vi "Set Parameter.vi"(4 "RingText.Text":string, 6 "txtpower":dbl, 7 "txtstepwave":dbl, 8 "error in":errorcluster, 9 "txtstopwave":dbl, 10 "txtstartwave":dbl, 11 "Address Cluster":T1 {"PCU_communcation_method" items=["GPIB", "C232C", "TCPIP", "USB"]; "tsl_communcation_method" items=["GPIB", "C232C", "TCPIP", "USB"]; "MPM_communcation_method" items=["GPIB", "C232C", "TCPIP", "USB"]}) -> (0 "error out":errorcluster, 3 "PDLSTS":refnum<k24>)   [LabVIEW 2017]
uses:
  CTL/Address Cluster.ctl
  D:/test/PDLSTS/LV_PDL_Sample/DLL/InstrumentDLL.dll
  DLL/InstrumentDLL.dll
  D:/test/PDLSTS/LV_PDL_Sample/DLL/STSProcess.dll
  DLL/STSProcess.dll
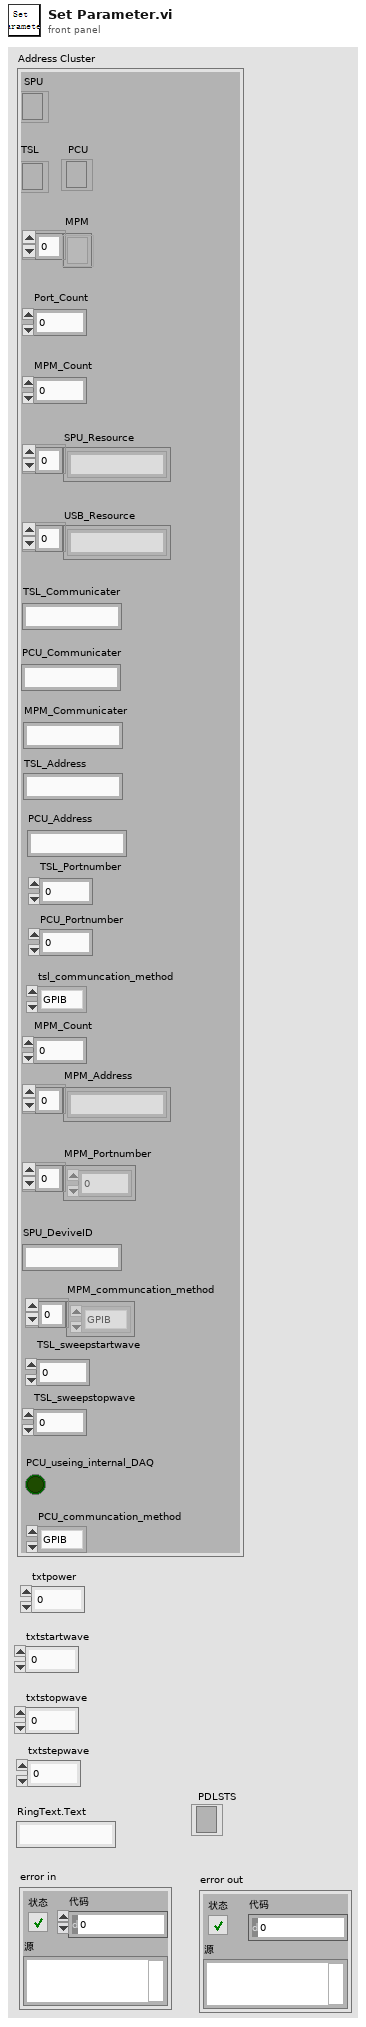
[diagram p1: front panel]
types:
  T1 = typedef "Address Cluster.ctl" = cluster{"SPU":refnum<k24>, "MPM":refnum<k24>[], "Port_Count":dbl, "MPM_Count":dbl, "SPU_Resource":string[], "USB_Resource":string[], "MPM_Communicater":string, "MPM_Count":dbl, "MPM_Address":string[], "MPM_Portnumber":dbl[], "SPU_DeviveID":string, "MPM_communcation_method":i32[], "TSL_sweepstartwave":dbl, "TSL_sweepstopwave":dbl, "TSL_Address":string, "TSL_Communicater":string, "TSL":refnum<k24>, "tsl_communcation_method":i32, "TSL_Portnumber":dbl, "PCU":refnum<k24>, "PCU_Communicater":string, "PCU_Address":string, "PCU_Portnumber":dbl, "PCU_useing_internal_DAQ":bool, "PCU_communcation_method":i32}
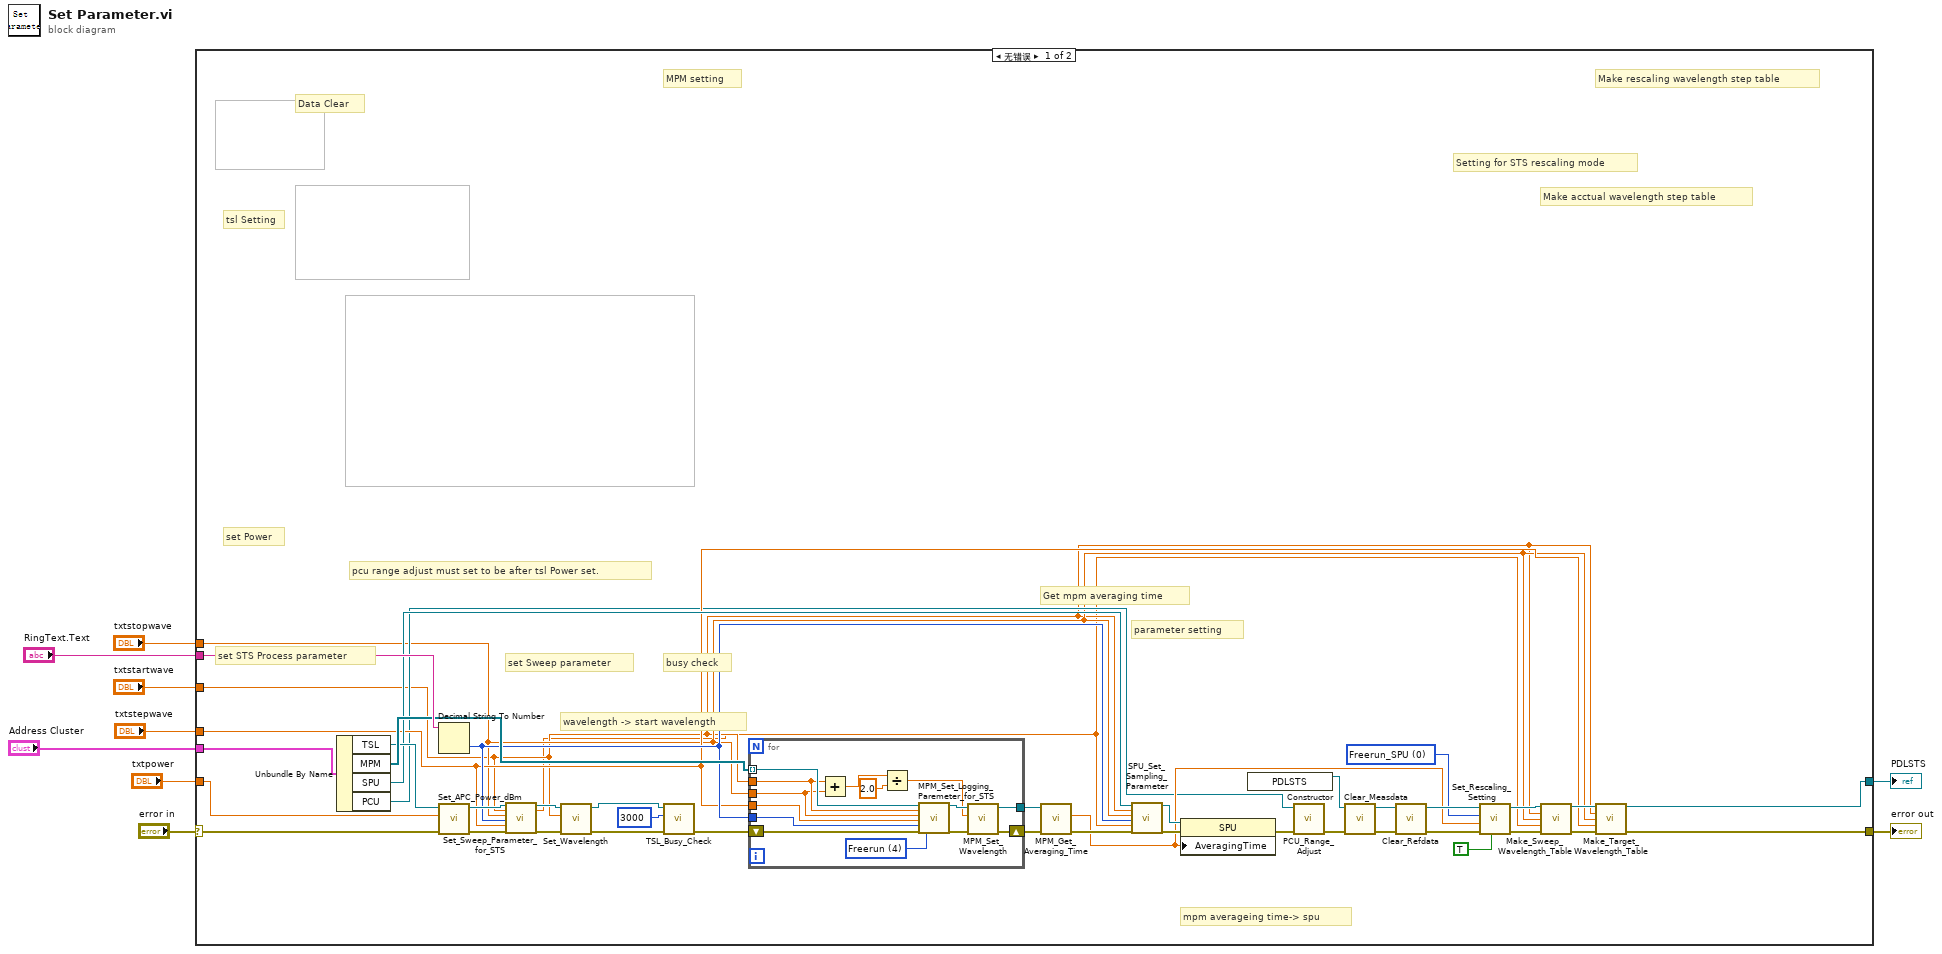
[diagram p0: block diagram]
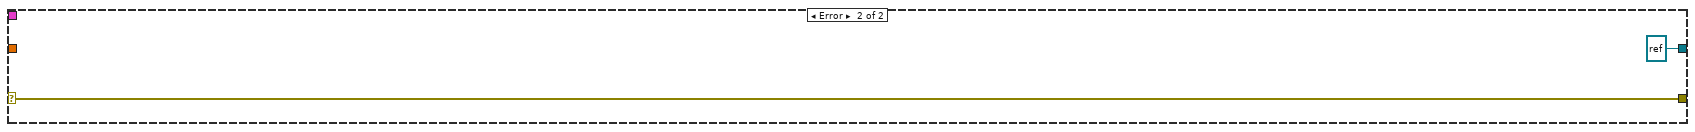
[diagram p2: hidden frame]
diagram:
  n1 = case shown="无错误" "error in" {
    selector: "error in" -> [w47 w67]
    tunnel: "txtstepwave" -> [w22 _]
    tunnel: "RingText.Text" -> [w51 _]
    tunnel: "txtpower" -> [w50 _]
    tunnel: [w13 refnum<k24> refnum ("Reference out")] -> w1
    tunnel: "Address Cluster" -> [w48 _]
    tunnel: [w46 w67] -> w4
    tunnel: "txtstopwave" -> [w12 _]
    tunnel: "txtstartwave" -> [w11 _]
    frame No Error {
      w36 = 0 items=["Freerun_SPU", "Freerun_Referencemodule"] ("mode")
      # "Make rescaling wavelength step table"
      # "Make acctual wavelength step table"
      # "Setting for STS rescaling mode"
      # "Data Clear"
      # "pcu range adjust must set to be after tsl Power set."
      # "mpm averageing time-> spu"
      # "parameter setting"
      # "Get mpm averaging time"
      # "MPM setting"
      # "busy check"
      # "set Sweep parameter"
      # "tsl Setting"
      # "set Power"
      # "set STS Process parameter"
      # "wavelength -> start wavelength"
      n2 = Unbundle By Name(w48) -> ("TSL"=w29:refnum<k24>, "MPM"=w49:refnum<k24>[], "SPU"=w25:refnum<k24>, "PCU"=w17:refnum<k24>)
      n3 = Decimal String To Number(string=w51) -> (number=w23:i32)  [unwired: 2 in, 1 out]
      n4 = call "Set_APC_Power_dBm.vi"(".NET Reference in"=w29, "Setting Power"=w50, "error in (no error)"=w47) -> ("Reference out"=w44:refnum<k24>, "error out"=w45:errorcluster)  [unwired: 6 in]
      n5 = call "Set_Sweep_Parameter_for_STS.vi"(".NET Reference in"=w44, "startwave"=w11, "stopwave"=w12, "speed"=w23, "rescalingstep"=w22, "error in (no error)"=w45) -> ("Reference out"=w43:refnum<k24>, "acctualstep"=w10:dbl, "error out"=w42:errorcluster)  [unwired: 11 in]
      n6 = call "Set_Wavelength.vi"("error in (no error)"=w42, "txtsetwave"=w11, ".NET Reference in"=w43) -> ("error out"=w28:errorcluster, "Reference out"=w21:refnum<k24>)  [unwired: 3 in]
      n7 = call "TSL_Busy_Check.vi"("error in (no error)"=w28, "Wait time(msec)"=3000, ".NET Reference in"=w21) -> ("error out"=w27:errorcluster)  [unwired: 7 in, 1 out]
      n8 = for {
        tunnel: w49 -> [w65] mode=indexing
        tunnel: w11 -> [w56]
        tunnel: w12 -> [w55]
        tunnel: w23 -> [w63]
        tunnel: w22 -> [w61]
        shift-right: [w59] -> w30
        shift-left: w27 -> [w64]
        tunnel: [w58] -> w31
        w62 = 4 items=["ManualRangeConstant", "ManualRangeSweep", "AutoRangeConstant", "AutoRangeSweep", "Freerun"] ("mode")
        n9 = Add(x=w56, y=w55) -> (x+y=w54:dbl)
        n10 = Divide(x=w54, y=2.0) -> (x/y=w52:dbl)
        n11 = call "MPM_Set_Logging_Paremeter_for_STS.vi"(".NET Reference in"=w65, "startwave"=w56, "stopwave"=w55, "wavestep"=w61, "speed"=w63, "error in (no error)"=w64, "mode"=w62) -> ("Reference out"=w57:refnum<k24>, "error out"=w60:errorcluster)  [unwired: 11 in]
        n12 = call "MPM_Set_Wavelength.vi"("error in (no error)"=w60, "Wavelength(nm)"=w52, ".NET Reference in"=w57) -> ("error out"=w59:errorcluster, "Reference out"=w58:refnum<k24>)  [unwired: 7 in]
      }
      n13 = call "MPM_Get_Averaging_Time.vi"("error in (no error)"=w30, ".NET Reference in"=w31) -> ("error out"=w24:errorcluster, "time out"=w18:dbl)  [unwired: 7 in, 1 out]
      n14 = call "SPU_Set_Sampling_Parameter.vi"("引用"=w25, "startwave"=w11, "stopwave"=w12, "speed"=w23, "triggerstep"=w10, "错误输入（无错误）"=w24) -> ("引用输出"=w20:refnum<k24>, "error IO"=w19:errorcluster)  [unwired: 12 in]
      n15 = property class="SPU"(reference=w20, error in=w19, "AveragingTime"=w18) -> (error out=w16:errorcluster)  [unwired: 1 out]
      n16 = constructor class="PDLSTS"() -> (reference out=w14:refnum<k24>)  [unwired: 3 in, 2 out]
      n17 = call "PCU_Range_Adjust.vi"("error in (no error)"=w16, ".NET Reference in"=w17) -> ("error out"=w15:errorcluster)  [unwired: 8 in, 1 out]
      n18 = call "Clear_Measdata.vi"("error in (no error)"=w15, ".NET Reference in"=w14) -> ("error out"=w40:errorcluster, "Reference out"=w41:refnum<k24>)  [unwired: 8 in]
      n19 = call "Clear_Refdata.vi"("error in (no error)"=w40, ".NET Reference in"=w41) -> ("error out"=w38:errorcluster, "Reference out"=w39:refnum<k24>)  [unwired: 8 in]
      n20 = call "Set_Rescaling_Setting.vi"("isOriginalMonitor"=TRUE, "error in (no error)"=w38, "avg"=w18, "mode"=w36, ".NET Reference in"=w39) -> ("error out"=w34:errorcluster, "Reference out"=w35:refnum<k24>)  [unwired: 5 in]
      n21 = call "Make_Sweep_Wavelength_Table.vi"(".NET Reference in"=w35, "startwave"=w11, "endwave"=w12, "triggerstep"=w10, "error in (no error)"=w34) -> ("Reference out"=w33:refnum<k24>, "error out"=w32:errorcluster)  [unwired: 9 in]
      n22 = call "Make_Target_Wavelength_Table.vi"(".NET Reference in"=w33, "startwave"=w11, "endwave"=w12, "targetdatastep"=w22, "error in (no error)"=w32) -> ("Reference out"=w13:refnum<k24>, "error out"=w46:errorcluster)  [unwired: 9 in]
    }
    frame Error {
    }
  }
  "error out" <- w4
  "PDLSTS" <- w1
